vi "pakage.vi"(8 "error in (no error)":errorcluster, 9 "Frame Instruction":T1, 10 "PN sequence order (9)":i32=9, 11 "text":string) -> (0 "error out":errorcluster, 3 "appended array":i8[](array[numeric]))   [LabVIEW 2014]
uses:
  <vilib>/addons/Modulation/Digital/General/MT Generate Bits (Galois, PN Order).vi
  <vilib>/addons/Modulation/Digital/Support/Common/Validators/mod_Generate Bits Validate.vi
  <vilib>/addons/Modulation/Analog/support/mod_Set Error Source.vi
  <vilib>/addons/Modulation/Digital/General/subVIs/mod_Generate Bits PN Sequence.vi
  <vilib>/addons/Modulation/niDMT.lvlib
panel:
  out "Numeric":dbl
  out "Array":i32[](array[numeric])
  out "message bitstream 2":i8[](array[numeric])
  out "Number of Packets":i32
  out "File Length (bits)":i32
  out "message bitstream":i8[](array[numeric])
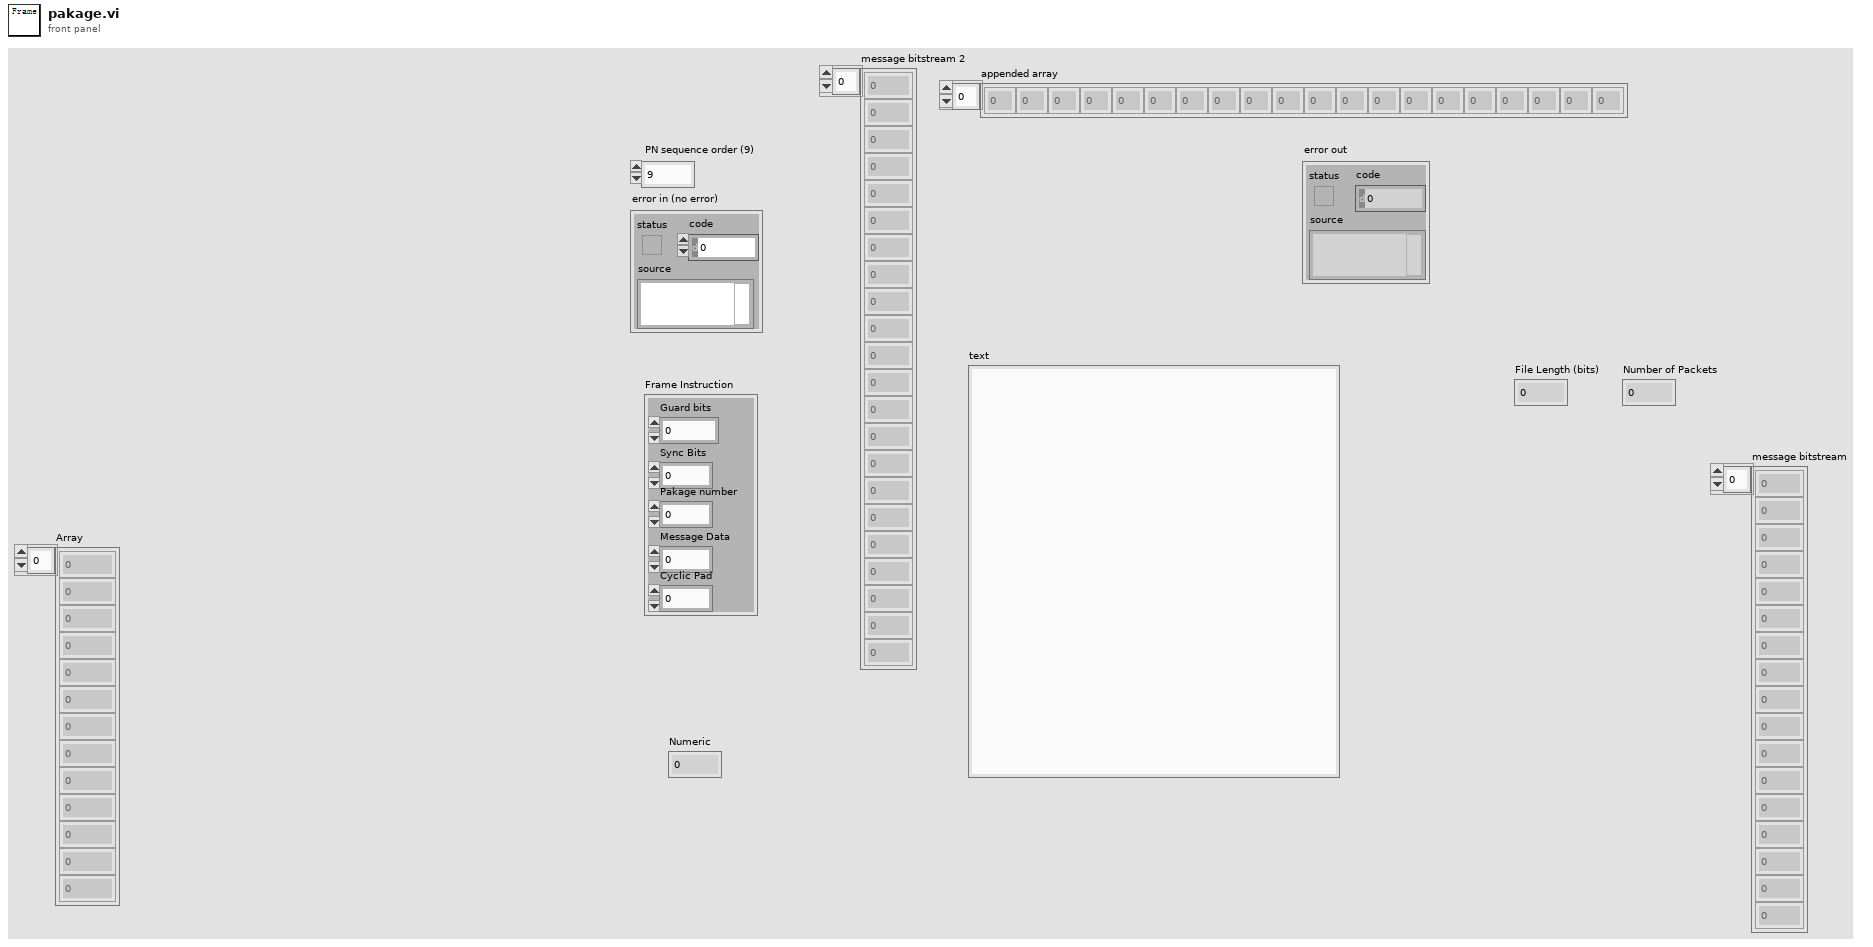
[diagram p1: front panel]
types:
  T1 = cluster{"Guard bits":dbl, "Sync Bits":dbl, "Pakage number":dbl, "Message Data":dbl, "Cyclic Pad":dbl}
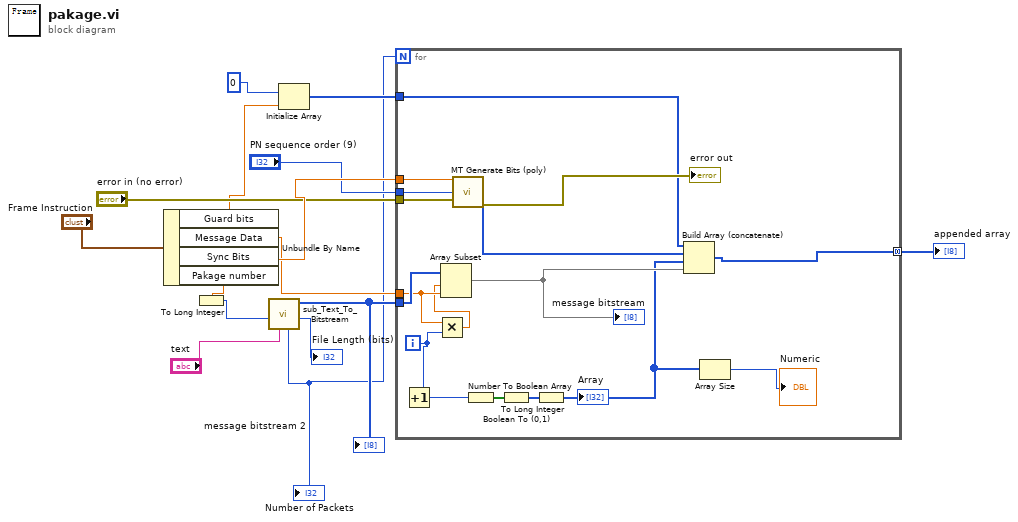
[diagram p0: block diagram]
diagram:
  n1 = Unbundle By Name("Frame Instruction") -> ("Guard bits"=w7:dbl, "Message Data"=w5:dbl, "Sync Bits"=w12:dbl)  [unwired: 1 out]
  n2 = To Long Integer(number=w5) -> (32bit integer=w2:i32)
  n3 = call "sub_Text_To_Bitstream.vi"("Packet\nMessage Length (bits)"=w2, "text"="text") -> ("File Length (bits)"=→"File Length (bits)":i32, "message bitstream"=w9:i8[], "Number of Packets"=w3:i32)  [unwired: 7 in]
  "Number of Packets" <- w3
  "message bitstream 2" <- w9
  n4 = Initialize Array(0, w7) -> (w6:i32[])
  n5 = for {
    N: w3 -> [_]
    tunnel: w12 -> [w31]
    tunnel: "PN sequence order (9)" -> [w30]
    tunnel: "error in (no error)" -> [w29]
    tunnel: w9 -> [w26]
    tunnel: w6 -> [w27]
    tunnel: w5 -> [w25]
    tunnel: [w23] -> w4 mode=concatenating
    i -> [w18]
    n6 = Increment(x=w18) -> (x+1=w21:i32)
    n7 = Multiply(x=w25, y=w18) -> (x*y=w24:dbl)
    n8 = Array Subset(array=w26, index=w24, length=w25) -> (w22:i8[])
    "message bitstream" <- w22
    n9 = call-poly <vilib>:"MT Generate Bits (poly).vi"("total bits (128)"=w31, "PN sequence order (9)"=w30, "error in (no error)"=w29) -> ("output bit stream"=w17:i8[], "error out"=→"error out":errorcluster)  [unwired: 10 in, 1 out]
    n10 = Number To Boolean Array(number=w21) -> (Boolean array=w20:bool[])
    n11 = Boolean To (0,1)(Boolean=w20) -> (0, 1=w19:i16[])
    n12 = To Long Integer(number=w19) -> (32bit integer=w16:i32[])
    "Array" <- w16
    n13 = Build Array (concatenate) "Build Array"(w27, w17, w16, w22) -> (w23:i32[])
    n14 = Array Size(array=w16) -> (size(s)=→"Numeric":i32)
  }
  "appended array" <- w4
